vi "Set Do Notifier.vi"(10 "Do Notifier":refnum<notifier>, 11 "Task Actor in":refnum<class "Task Actor.lvclass">) -> (3 "Task Actor out":refnum<class "Task Actor.lvclass">)   [LabVIEW 2025, in "Task Actor.lvlib" / "Task Actor.lvclass"]
uses:
  Task Actor.lvclass
  <vilib>/ActorFramework/Time-Delayed Send Message/Time-Delay Override Options.ctl
  Task Actor.lvclass/Task Actor.ctl
  <vilib>/ActorFramework/Actor Framework.lvlib
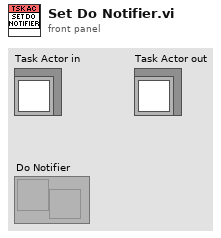
[diagram p1: front panel]
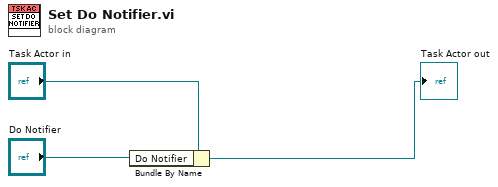
[diagram p0: block diagram]
diagram:
  n1 = Bundle By Name(cluster="Task Actor in", "Do Notifier"="Do Notifier") -> (→"Task Actor out":refnum<class "Task Actor.lvclass">)
